vi "TwoBendingRootSubVi.vi"(0 "x node":i32, 1 "y node":i32, 2 "t":dbl, 3 "u":dbl, 4 "amp 1":dbl, 5 "amp 2":dbl, 6 "x":dbl, 7 "nL":dbl, 9 "phi 1":dbl, 11 "phi 2":dbl) -> (14 "BendRoot":dbl, 19 "Bend":dbl)   [LabVIEW 2017]
panel:
  # "Salmon Parameters (amp1 = 0.0488,amp2 = 0.0832,phi=0.8499,c=0.0281,u=62.8319)"
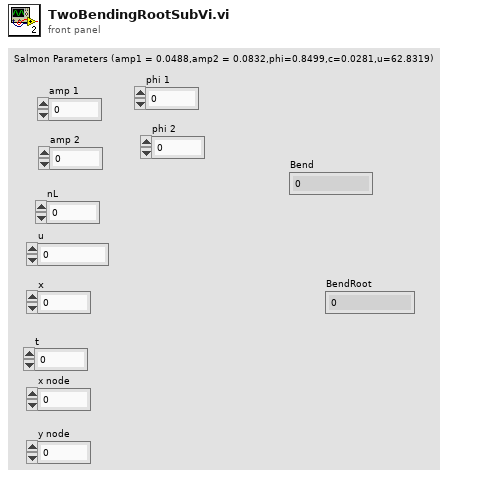
[diagram p1: front panel]
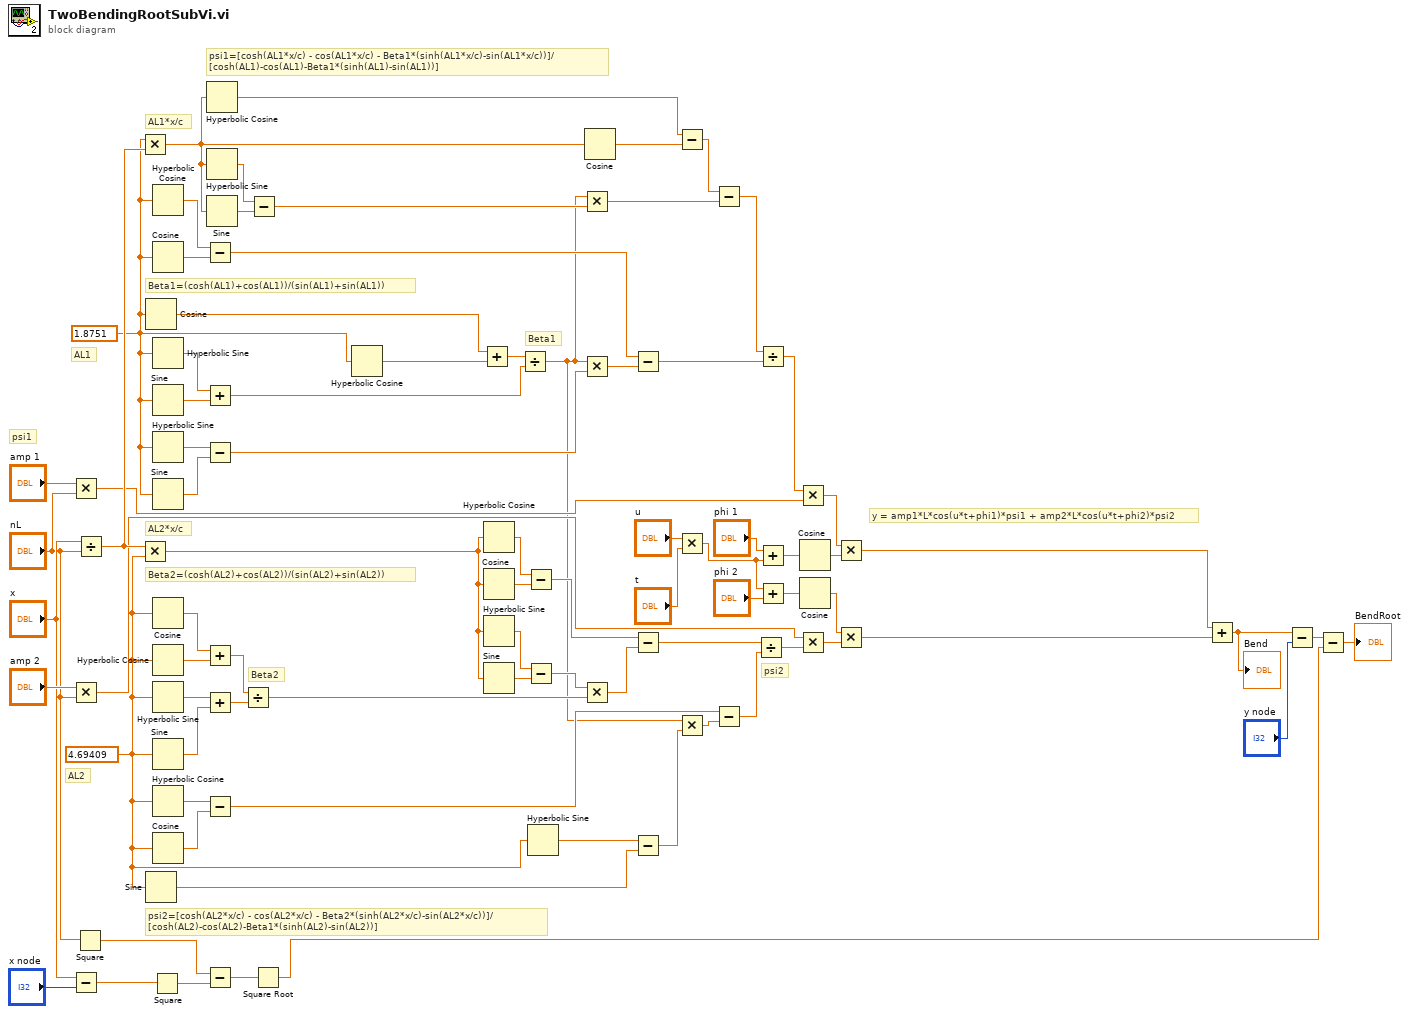
[diagram p0: block diagram]
diagram:
  w33 = 4.69409
  w60 = 1.8751
  # "psi2"
  # "psi1"
  # "AL2*x/c"
  # "AL1*x/c"
  # "psi2=[cosh(AL2*x/c) - cos(AL2*x/c) - Beta2*(sinh(AL2*x/c)-sin(AL2*x/c))]/\n[cosh(AL2)-cos(AL2)-Beta1*(sinh(AL2)-sin(AL2))]"
  # "psi1=[cosh(AL1*x/c) - cos(AL1*x/c) - Beta1*(sinh(AL1*x/c)-sin(AL1*x/c))]/\n[cosh(AL1)-cos(AL1)-Beta1*(sinh(AL1)-sin(AL1))]"
  # "y = amp1*L*cos(u*t+phi1)*psi1 + amp2*L*cos(u*t+phi2)*psi2"
  # "Beta2=(cosh(AL2)+cos(AL2))/(sin(AL2)+sin(AL2))"
  # "Beta1=(cosh(AL1)+cos(AL1))/(sin(AL1)+sin(AL1))"
  # "Beta2"
  # "Beta1"
  # "AL2"
  # "AL1"
  n1 = Multiply(x="amp 1", y="nL") -> (x*y=w45:dbl)
  n2 = Multiply(x="amp 2", y="nL") -> (x*y=w22:dbl)
  n3 = Subtract(x="x", y="x node") -> (x-y=w9:dbl)
  n4 = Square(x="nL") -> (x^2=w6:dbl)
  n5 = Divide(x="x", y="nL") -> (x/y=w70:dbl)
  n6 = Multiply(x=w60, y=w70) -> (x*y=w69:dbl)
  n7 = Multiply(x=w70, y=w33) -> (x*y=w34:dbl)
  n8 = Cosine(x=w60) -> (cos(x)=w81:dbl)
  n9 = Sine(x=w33) -> (sin(x)=w35:dbl)
  n10 = Square(x=w9) -> (x^2=w5:dbl)
  n11 = Hyperbolic Cosine(1:w60) -> (0:w59:dbl)
  n12 = Cosine(x=w60) -> (cos(x)=w58:dbl)
  n13 = Hyperbolic Sine(1:w60) -> (0:w80:dbl)
  n14 = Sine(x=w60) -> (sin(x)=w79:dbl)
  n15 = Hyperbolic Sine(1:w60) -> (0:w57:dbl)
  n16 = Sine(x=w60) -> (sin(x)=w56:dbl)
  n17 = Cosine(x=w33) -> (cos(x)=w77:dbl)
  n18 = Hyperbolic Cosine(1:w33) -> (0:w78:dbl)
  n19 = Hyperbolic Sine(1:w33) -> (0:w76:dbl)
  n20 = Sine(x=w33) -> (sin(x)=w75:dbl)
  n21 = Hyperbolic Cosine(1:w33) -> (0:w38:dbl)
  n22 = Cosine(x=w33) -> (cos(x)=w37:dbl)
  n23 = Subtract(x=w59, y=w58) -> (x-y=w53:dbl)
  n24 = Add(x=w80, y=w79) -> (x+y=w73:dbl)
  n25 = Subtract(x=w57, y=w56) -> (x-y=w55:dbl)
  n26 = Add(x=w77, y=w78) -> (x+y=w72:dbl)
  n27 = Add(x=w76, y=w75) -> (x+y=w71:dbl)
  n28 = Subtract(x=w38, y=w37) -> (x-y=w16:dbl)
  n29 = Subtract(x=w6, y=w5) -> (x-y=w7:dbl)
  n30 = Hyperbolic Cosine(1:w69) -> (0:w65:dbl)
  n31 = Hyperbolic Sine(1:w69) -> (0:w68:dbl)
  n32 = Sine(x=w69) -> (sin(x)=w67:dbl)
  n33 = Divide(x=w72, y=w71) -> (x/y=w28:dbl)
  n34 = Subtract(x=w68, y=w67) -> (x-y=w66:dbl)
  n35 = Square Root(x=w7) -> (sqrt(x)=w4:dbl)
  n36 = Hyperbolic Cosine(1:w60) -> (0:w82:dbl)
  n37 = Add(x=w81, y=w82) -> (x+y=w74:dbl)
  n38 = Hyperbolic Cosine(1:w34) -> (0:w40:dbl)
  n39 = Cosine(x=w34) -> (cos(x)=w39:dbl)
  n40 = Hyperbolic Sine(1:w34) -> (0:w42:dbl)
  n41 = Sine(x=w34) -> (sin(x)=w41:dbl)
  n42 = Divide(x=w74, y=w73) -> (x/y=w13:dbl)
  n43 = Subtract(x=w40, y=w39) -> (x-y=w19:dbl)
  n44 = Subtract(x=w42, y=w41) -> (x-y=w27:dbl)
  n45 = Hyperbolic Sine(1:w33) -> (0:w36:dbl)
  n46 = Multiply(x=w13, y=w66) -> (x*y=w62:dbl)
  n47 = Multiply(x=w13, y=w55) -> (x*y=w54:dbl)
  n48 = Multiply(x=w27, y=w28) -> (x*y=w18:dbl)
  n49 = Cosine(x=w69) -> (cos(x)=w64:dbl)
  n50 = Subtract(x=w53, y=w54) -> (x-y=w52:dbl)
  n51 = Subtract(x=w19, y=w18) -> (x-y=w17:dbl)
  n52 = Subtract(x=w36, y=w35) -> (x-y=w15:dbl)
  n53 = Subtract(x=w65, y=w64) -> (x-y=w63:dbl)
  n54 = Multiply(x="u", y="t") -> (x*y=w32:dbl)
  n55 = Multiply(x=w13, y=w15) -> (x*y=w14:dbl)
  n56 = Subtract(x=w63, y=w62) -> (x-y=w61:dbl)
  n57 = Subtract(x=w16, y=w14) -> (x-y=w20:dbl)
  n58 = Divide(x=w17, y=w20) -> (x/y=w21:dbl)
  n59 = Divide(x=w61, y=w52) -> (x/y=w46:dbl)
  n60 = Add(x="phi 1", y=w32) -> (x+y=w47:dbl)
  n61 = Add(x=w32, y="phi 2") -> (x+y=w29:dbl)
  n62 = Multiply(x=w46, y=w45) -> (x*y=w44:dbl)
  n63 = Multiply(x=w22, y=w21) -> (x*y=w23:dbl)
  n64 = Cosine(x=w47) -> (cos(x)=w43:dbl)
  n65 = Cosine(x=w29) -> (cos(x)=w24:dbl)
  n66 = Multiply(x=w44, y=w43) -> (x*y=w26:dbl)
  n67 = Multiply(x=w24, y=w23) -> (x*y=w25:dbl)
  n68 = Add(x=w26, y=w25) -> (x+y=w1:dbl)
  "Bend" <- w1
  n69 = Subtract(x=w1, y="y node") -> (x-y=w10:dbl)
  n70 = Subtract(x=w10, y=w4) -> (x-y=→"BendRoot":dbl)
